vi "gesty.vi"(6 "Przyciski":u8[](array[numeric]), 7 "Kanały serwa":u8[](array[numeric]), 8 "zatrzymanie wybierania gestów":bool, 9 "LINX SERWO":T1, 10 "Error In":errorcluster, 11 "DIGITAL READ":T1) -> ()   [LabVIEW 2025]
doc: "Use this template to build a standard state machine design pattern. Each state executes code and determines which state to transition to. Contrast this design pattern with the User Interface Event Handler pattern, in which code executes in response to user actions. Contrast this design pattern also with the Queued Message Handler pattern, in which each message handling code can queue zero or more new messages.\nNote: This template does not contain the most recent programming guidelines recommended by National Instruments. For a complete, project-based implementation of the Standard State Machine pattern, use the Create Project dialog box instead of this template."
uses:
  <vilib>/MakerHub/LINX/Private/Type Defs/LINX Ref.ctl
  <vilib>/MakerHub/LINX/Private/Type Defs/Platform.ctl
  <vilib>/MakerHub/LINX/Private/Type Defs/Interface.ctl
  <vilib>/MakerHub/LINX/Private/Device/Type Defs/LINX Device Config.ctl
  <vilib>/MakerHub/LINX/Private/Device/Type Defs/TCP Config.ctl
  <vilib>/MakerHub/LINX/Private/Device/Type Defs/Channels.ctl
  <vilib>/MakerHub/LINX/Public/Peripherals/Digital/Digital Read N Chans.vi
  <vilib>/MakerHub/LINX/Private/Local IO/LinxDigitalRead.vi
  <vilib>/MakerHub/LINX/Public/Utilities/Check Channel.vi
  <vilib>/MakerHub/LINX/Private/Utilties/Generate Error.vi
  <vilib>/MakerHub/LINX/Public/Sensors/Motion/Servo/Servo Set Pulse Width N Channels.vi
  <vilib>/MakerHub/LINX/Public/Sensors/Motion/Servo/Servo.lvlib
  <vilib>/MakerHub/LINX/LMH-LINX.lvlib
  <vilib>/MakerHub/LINX/Private/Device/Device.lvlib
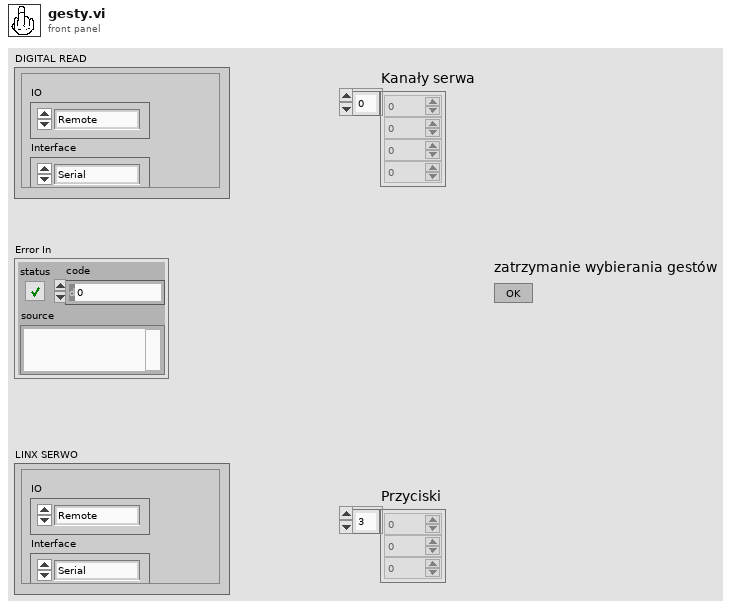
[diagram p1: front panel]
types:
  T1 = typedef "LMH-LINX.lvlib/LINX Ref.ctl" = cluster{"IO":T2, "Interface":T3, "LINX Device Config":T4}
  T2 = typedef "LMH-LINX.lvlib/Platform.ctl" = enum16{"Remote", "Local"}
  T3 = typedef "LMH-LINX.lvlib/Interface.ctl" = enum16{"Serial", "TCP"}
  T4 = typedef "LMH-LINX.lvlib/Device.lvlib/LINX Device Config.ctl" = cluster{"Interface":T3, "COM Port":refnum<visa-resource-name>, "TCP Configuration":T5, "Device Family":u8, "Device ID":u8, "Device Name":string, "TCP Ref":refnum<k5>, "Channels":T6}
  T5 = typedef "LMH-LINX.lvlib/Device.lvlib/TCP Config.ctl" = cluster{"IP Address":string, "Port":u16}
  T6 = typedef "LMH-LINX.lvlib/Channels.ctl" = cluster{"DI":u8[], "DO":u8[], "AI":u8[], "AO":u8[], "PWM":u8[], "QE":u8[], "UART":u8[], "I2C 2":u8[], "SPI":u8[], "CAN":u8[], "Servo":u8[], "AI Ref (V)":dbl, "AI Resolution (Bits)":u8, "AO Ref (V)":dbl, "AO Resolution (Bits)":u8}
  T7 = typedef "kontrolaGestów.ctt" = enum16{"wybierz", "rewolwer", "rock and roll", "faker nie raper", "dwa palce w natalce", "Initialize", "Stop"}
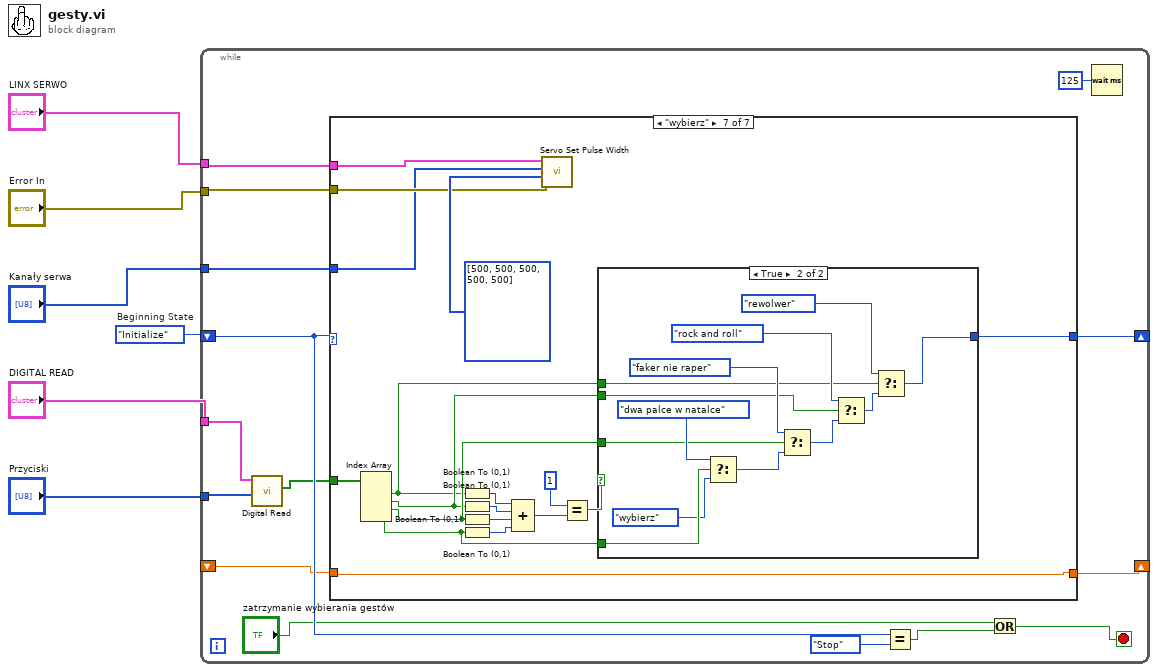
[diagram p0: block diagram]
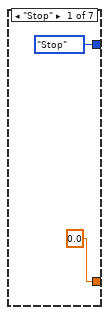
[diagram p2: hidden frame]
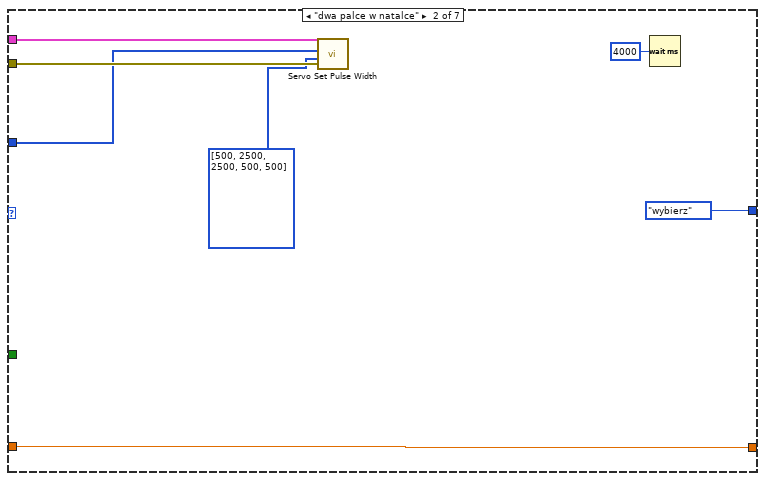
[diagram p3: hidden frame]
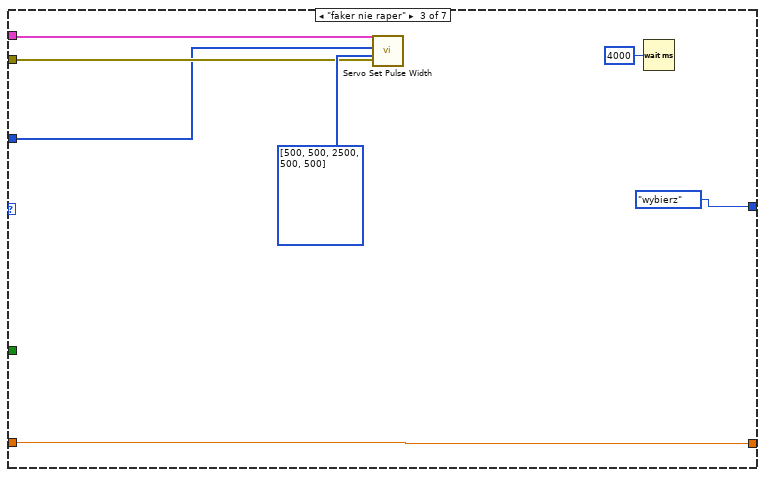
[diagram p4: hidden frame]
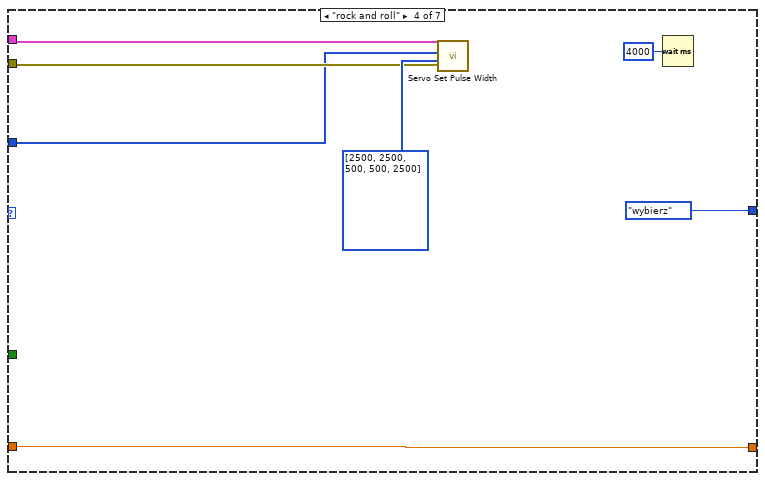
[diagram p5: hidden frame]
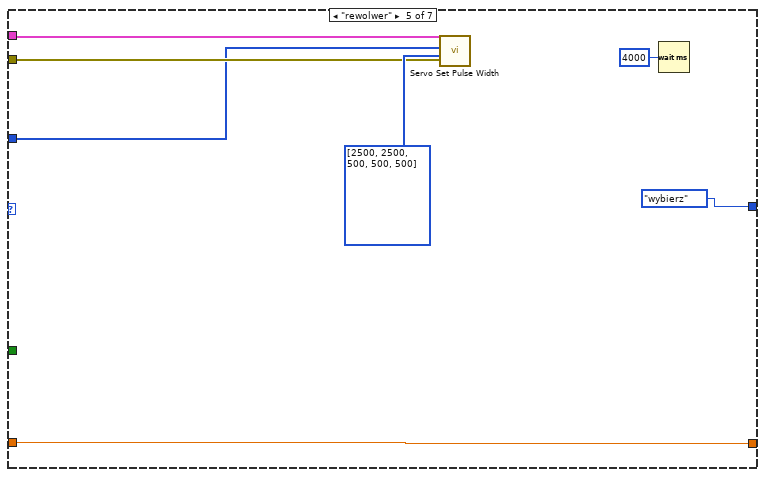
[diagram p6: hidden frame]
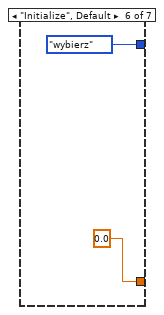
[diagram p7: hidden frame]
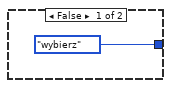
[diagram p8: hidden frame]
diagram:
  w6 = kontrolaGestów.ctt."Initialize"  # Beginning State
  n1 = while {
    shift-right: [w19] -> _
    shift-left: w6 -> [w20]
    tunnel: "LINX SERWO" -> [w17]
    tunnel: "Error In" -> [w16]
    tunnel: "DIGITAL READ" -> [w15]
    tunnel: "Przyciski" -> [w14]
    shift-right: [w12] -> _
    shift-left: _ -> [w11]
    tunnel: "Kanały serwa" -> [w10]
    stop <- w7 stop-if-true
    n2 = call-poly <vilib>:"Digital Read.vi"("DI Channels"=w14, "LINX Resource"=w15) -> ("Values"=w13:bool[])  [unwired: 7 in, 2 out]
    n3 = case shown="\"wybierz\"" w20 {
      tunnel: [kontrolaGestów.ctt."Stop" ("Next State") kontrolaGestów.ctt."wybierz" ("States") kontrolaGestów.ctt."wybierz" ("States") kontrolaGestów.ctt."wybierz" ("States") kontrolaGestów.ctt."wybierz" ("States") kontrolaGestów.ctt."wybierz" ("States") w67] -> w19
      tunnel: w17 -> [_ w30 w36 w43 w49 _ w56]
      tunnel: w16 -> [_ w29 w35 w42 w48 _ w55]
      tunnel: w13 -> [_ _ _ _ _ _ w71]
      tunnel: [0.0 w26 w33 w39 w51 0.0 w58] -> w12
      tunnel: w11 -> [_ w26 w33 w39 w51 _ w58]
      tunnel: w10 -> [_ w24 w31 w40 w45 _ w54]
      frame "Stop" {
      }
      frame "dwa palce w natalce" {
        n4 = call-poly <vilib>:"Servo Set Pulse Width.vi"("Error In"=w29, "Pulse Widths (uS)"=u16[] [500, 2500, 2500, 500, 500], "Servo Channels"=w24, "LINX Resource"=w30) -> ()  [unwired: 6 in, 2 out]
        n5 = Wait (ms)(milliseconds to wait=u32 4000) -> ()  [unwired: 1 out]
      }
      frame "faker nie raper" {
        n6 = call-poly <vilib>:"Servo Set Pulse Width.vi"("Error In"=w35, "Pulse Widths (uS)"=u16[] [500, 500, 2500, 500, 500], "Servo Channels"=w31, "LINX Resource"=w36) -> ()  [unwired: 6 in, 2 out]
        n7 = Wait (ms)(milliseconds to wait=u32 4000) -> ()  [unwired: 1 out]
      }
      frame "rock and roll" {
        n8 = call-poly <vilib>:"Servo Set Pulse Width.vi"("Error In"=w42, "Pulse Widths (uS)"=u16[] [2500, 2500, 500, 500, 2500], "Servo Channels"=w40, "LINX Resource"=w43) -> ()  [unwired: 6 in, 2 out]
        n9 = Wait (ms)(milliseconds to wait=u32 4000) -> ()  [unwired: 1 out]
      }
      frame "rewolwer" {
        n10 = call-poly <vilib>:"Servo Set Pulse Width.vi"("Error In"=w48, "Pulse Widths (uS)"=u16[] [2500, 2500, 500, 500, 500], "Servo Channels"=w45, "LINX Resource"=w49) -> ()  [unwired: 6 in, 2 out]
        n11 = Wait (ms)(milliseconds to wait=u32 4000) -> ()  [unwired: 1 out]
      }
      frame "Initialize", Default {
      }
      frame "wybierz" {
        n12 = Index Array(array=w71) -> (element #1=w59:bool, element #2=w60:bool, element #3=w61:bool, element #4=w62:bool)  [unwired: 4 in]
        n13 = Boolean To (0,1)(Boolean=w59) -> (0, 1=w66:i16)
        n14 = Boolean To (0,1)(Boolean=w60) -> (0, 1=w65:i16)
        n15 = Boolean To (0,1)(Boolean=w61) -> (0, 1=w64:i16)
        n16 = Boolean To (0,1)(Boolean=w62) -> (0, 1=w63:i16)
        n17 = Compound Arithmetic op=ADD(w66, w65, w64, w63) -> (w70:i16)
        n18 = call-poly <vilib>:"Servo Set Pulse Width.vi"("Error In"=w55, "Pulse Widths (uS)"=u16[] [500, 500, 500, 500, 500], "Servo Channels"=w54, "LINX Resource"=w56) -> ()  [unwired: 6 in, 2 out]
        n19 = Equal?(x=i16 1, y=w70) -> (x = y?=w68:bool)
        n20 = case shown="True" w68 {
          tunnel: [kontrolaGestów.ctt."wybierz" ("States") w76] -> w67
          tunnel: w62 -> [_ w85]
          tunnel: w61 -> [_ w75]
          tunnel: w60 -> [_ w74]
          tunnel: w59 -> [_ w73]
          frame False {
          }
          frame True {
            n21 = Select(t=kontrolaGestów.ctt."dwa palce w natalce" ("States"), s=w85, f=kontrolaGestów.ctt."wybierz" ("States")) -> (s? t:f=w79:T7)
            n22 = Select(t=kontrolaGestów.ctt."faker nie raper" ("States"), s=w75, f=w79) -> (s? t:f=w78:T7)
            n23 = Select(t=kontrolaGestów.ctt."rock and roll" ("States"), s=w74, f=w78) -> (s? t:f=w77:T7)
            n24 = Select(t=kontrolaGestów.ctt."rewolwer" ("States"), s=w73, f=w77) -> (s? t:f=w76:T7)
          }
        }
      }
    }
    n25 = Equal?(x=w20, y=kontrolaGestów.ctt."Stop" ("States")) -> (x = y?=w8:bool)
    n26 = Or(x="zatrzymanie wybierania gestów", y=w8) -> (x .or. y?=w7:bool)
    n27 = Wait (ms)(milliseconds to wait=u32 125) -> ()  [unwired: 1 out]
  }
